vi "Translate ByRef.vi"(8 "error in (no error)":errorcluster, 10 "Translation":T1, 11 "ShapeRef":refnum<data-value>) -> (0 "error out":errorcluster, 3 "ShapeRef Out":refnum<data-value>)   [LabVIEW 2015, in "LV Image Editor Framework.lvlib" / "Shape.lvclass"]
uses:
  Shape.lvclass
  <vilib>/Utility/miscctls.llb/LVPoint32TypeDef.ctl
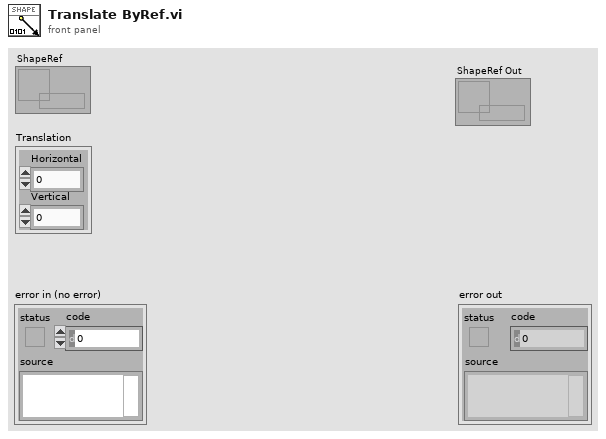
[diagram p1: front panel]
types:
  T1 = typedef "LVPoint32TypeDef.ctl" = cluster{"Horizontal":i32, "Vertical":i32}
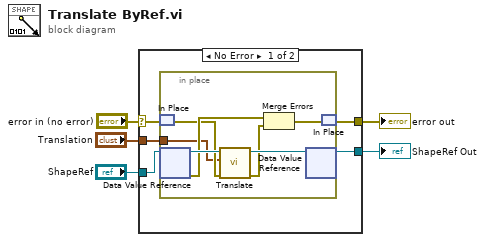
[diagram p0: block diagram]
diagram:
  n1 = case shown="No Error" "error in (no error)" {
    selector: "error in (no error)" -> [w8 w19]
    tunnel: [w7 w19] -> w4
    tunnel: "ShapeRef" -> [w10 w18]
    tunnel: [w9 w18] -> w2
    tunnel: "Translation" -> [w6 _]
    frame No Error {
      n2 = in-place {
        in-place-border: w6 -> [w11]
        n3 = in-place-match #1(w8) -> (w13:errorcluster)
        n4 = in-place-dvr #2(w10) -> (w16:refnum<class "Shape.lvclass">, w15:errorcluster)
        n5 = call "Translate.vi"("error in (no error)"=w13, "Translation"=w11, "Shape in"=w16) -> ("error out"=w14:errorcluster, "Shape out"=w17:refnum<class "Shape.lvclass">)  [unwired: 7 in]
        n6 = Merge Errors(w15, w14) -> (w12:errorcluster)
        n7 = in-place-dvr #2(w17) -> (w9:refnum<data-value>)  [unwired: 1 out]
        n8 = in-place-match #1(w12) -> (w7:errorcluster)
      }
    }
    frame Error {
    }
  }
  "error out" <- w4
  "ShapeRef Out" <- w2
